vi "visualization.vi"() -> ()   [LabVIEW 2024]
uses:
  <vilib>/Analysis/baseanly.llb/Mean (DBL).vi
  <vilib>/picture/3D Picture Control/Object/Create Object (name).vi
  <vilib>/Utility/file.llb/Read Delimited Spreadsheet (string).vi
  <vilib>/picture/3D Picture Control/Helpers/Set Light (no reference).vi
  <vilib>/picture/3D Picture Control/NI_3D Picture Control.lvlib
  <vilib>/Analysis/NI_AALBase.lvlib
panel:
  out "XY Graph 4":cluster{dbl[], dbl[]}[](graph)
  out "XY Graph 3":cluster{dbl[], dbl[]}[](graph)
  out "XY Graph 2":cluster{dbl[], dbl[]}[](graph)
  out "XY Graph":cluster{dbl[], dbl[]}[](graph)
  out "Slide":u8(slide) scale=0.0..100.0
  in  "stop":bool
  out "3D Picture 2":refnum<vi>(3d-picture)
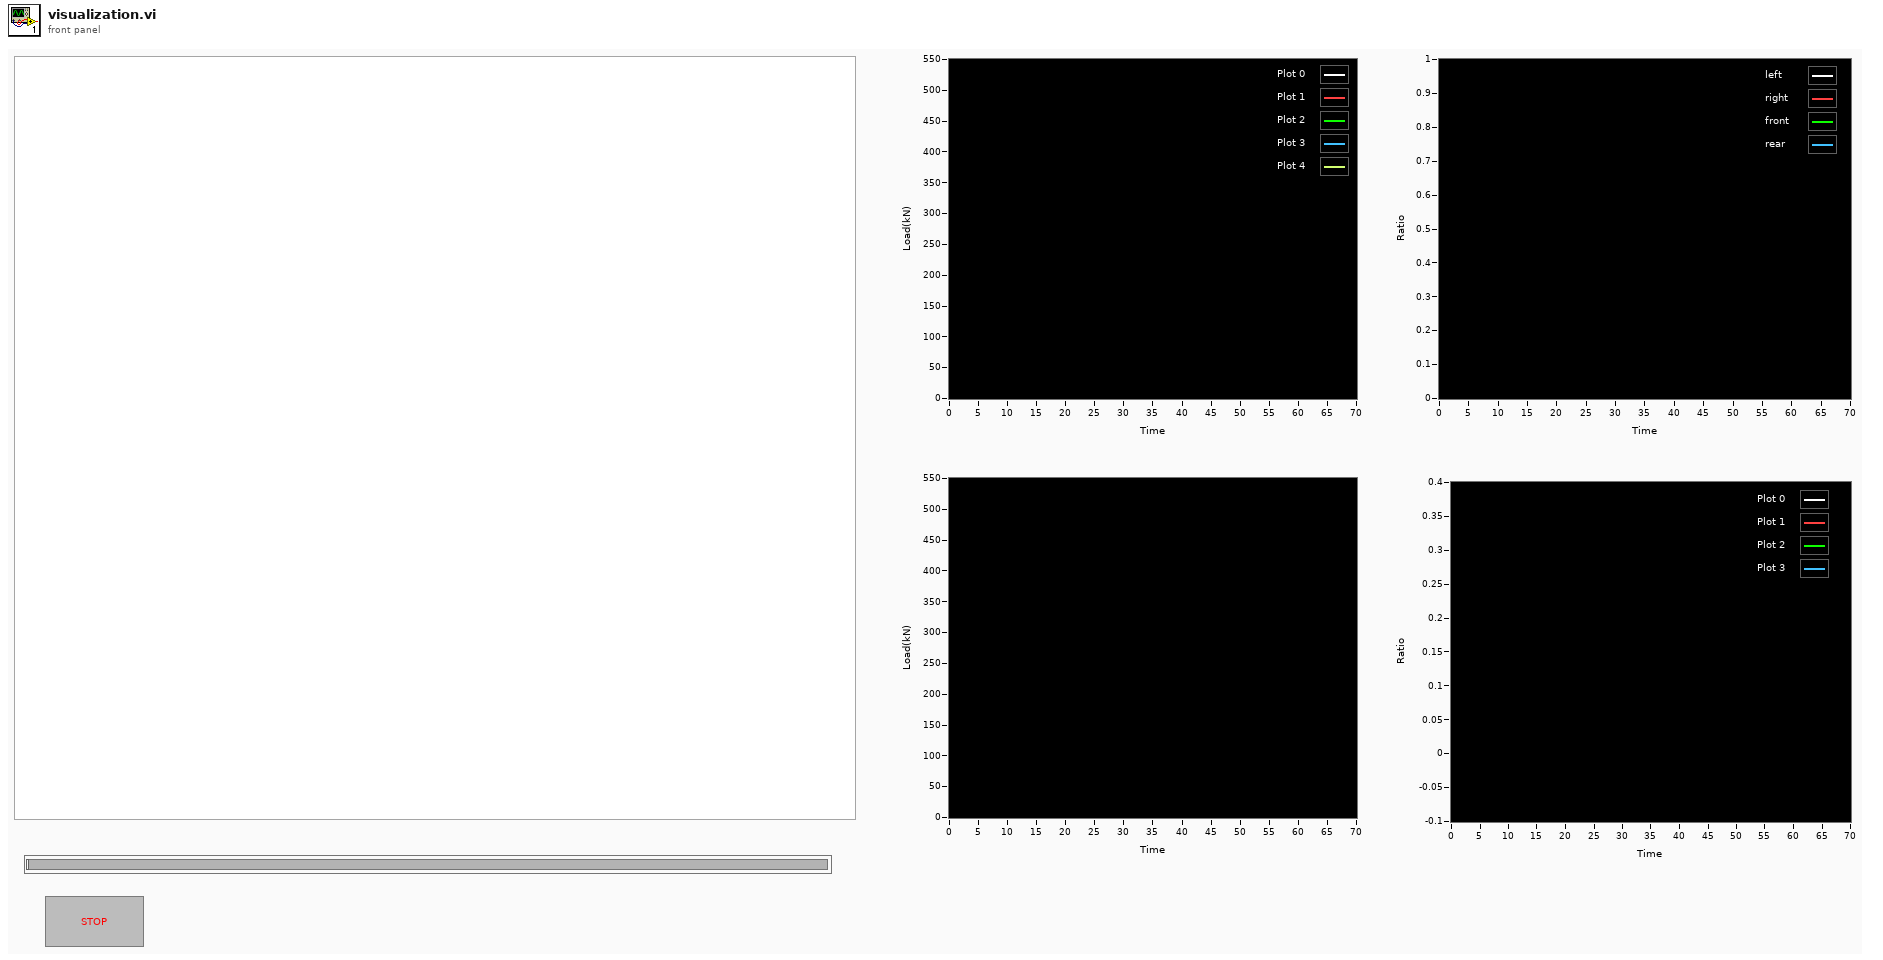
[diagram p1: front panel]
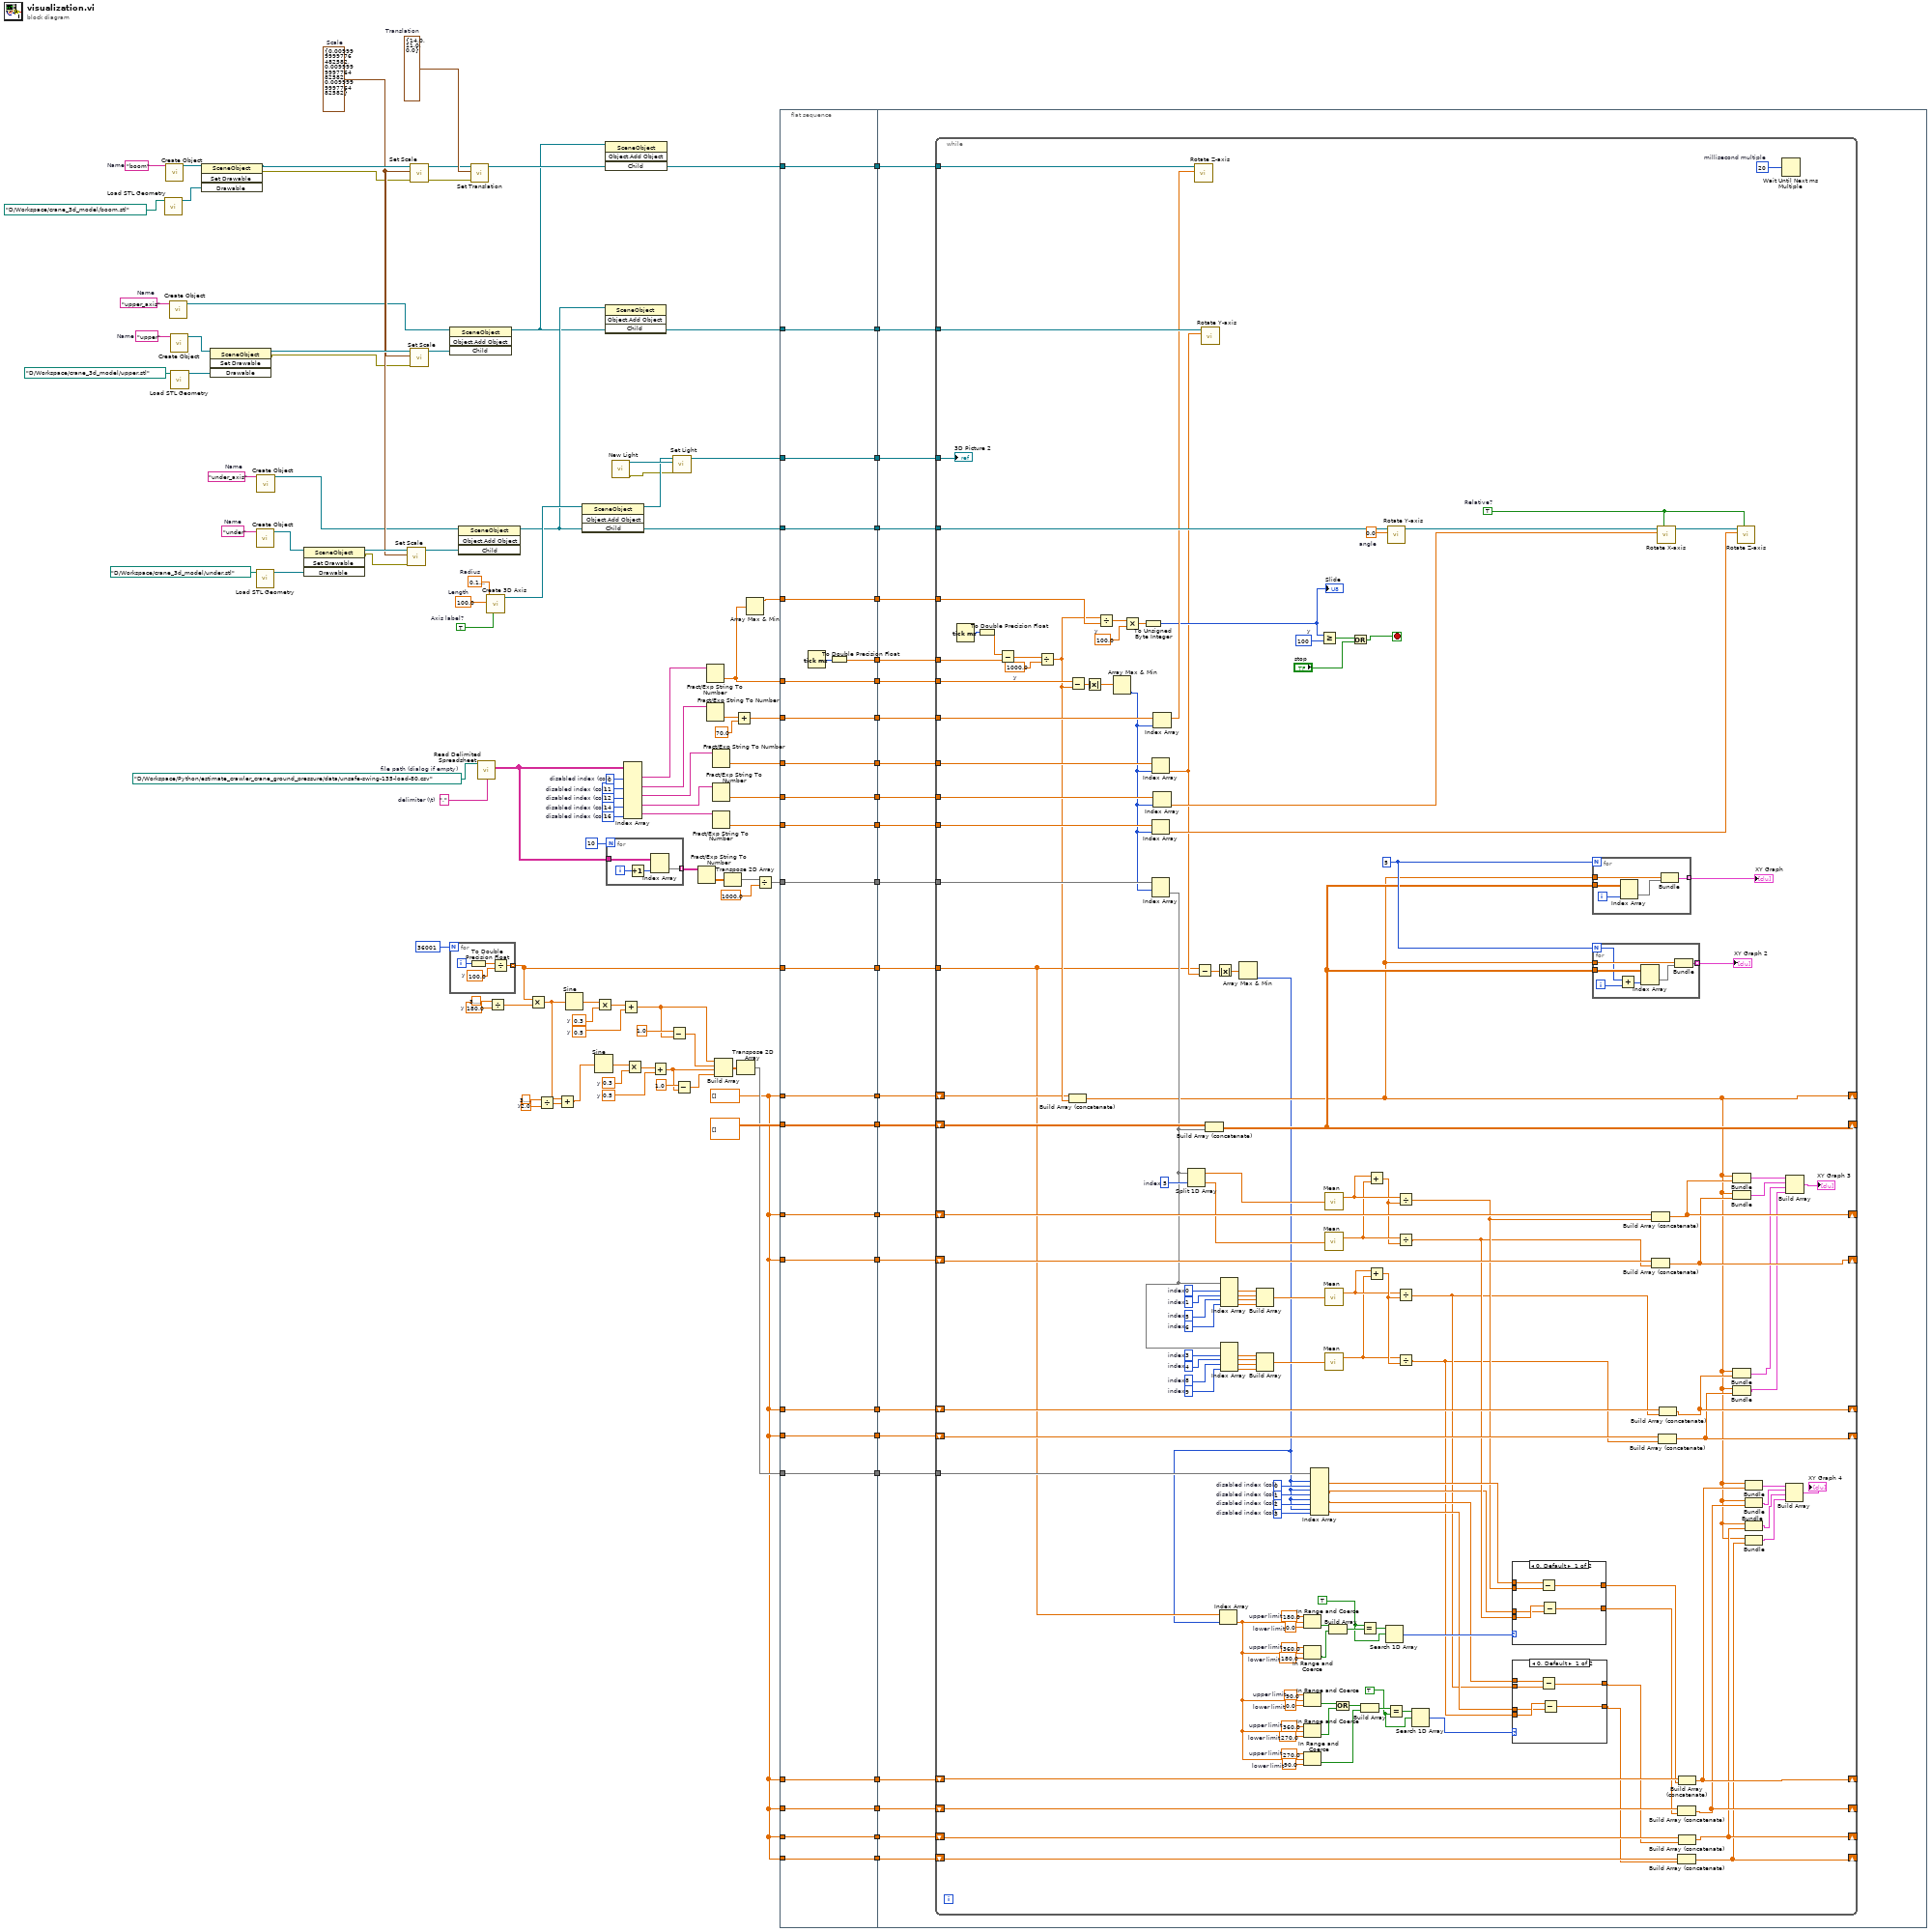
[diagram p0: block diagram]
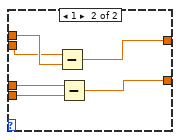
[diagram p2: hidden frame]
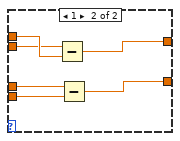
[diagram p3: hidden frame]
diagram:
  w7 = 0.5  # y
  w8 = 0.5  # y
  w15 = 0.3  # y
  w19 = 2.0  # y
  w29 = 0.3  # y
  w33 = 180.0  # y
  w1 = dbl[] []
  w66 = 16  # disabled index (col)
  w67 = 14  # disabled index (col)
  w71 = 12  # disabled index (col)
  w76 = 11  # disabled index (col)
  w77 = 0  # disabled index (col)
  w78 = ","  # delimiter (\t)
  w79 = path "D:/Workspace/Python/estimate_crawler_crane_ground_pressure/data/unsafe-swing-135-load-80.csv"  # file path (dialog if empty)
  w90 = "upper_axis"  # Name
  w92 = "under_axis"  # Name
  w102 = cluster{"X":sgl, "Y":sgl, "Z":sgl} {"X"=14.0, "Y"=11.0, "Z"=0.0}  # Translation
  w100 = cluster{"X":sgl, "Y":sgl, "Z":sgl} {"X"=0.01, "Y"=0.01, "Z"=0.01}  # Scale
  w104 = "under"  # Name
  w109 = "upper"  # Name
  w113 = sgl 0.1  # Radius
  w116 = sgl 100.0  # Length
  w118 = TRUE  # Axis label?
  w119 = "boom"  # Name
  n1 = call <vilib>:"Load STL Geometry.vi"("Model File"=path "D:/Workspace/crane_3d_model/boom.stl") -> ("New Mesh Refnum"=w117:refnum<vi>)  [unwired: 9 in, 1 out]
  n2 = call-poly <vilib>:"Create Object.vi"("Name"=w119) -> ("Scene:New Object"=w120:refnum<vi>)  [unwired: 9 in, 1 out]
  n3 = call-poly <vilib>:"Create Object.vi"("Name"=w90) -> ("Scene:New Object"=w88:refnum<vi>)  [unwired: 9 in, 1 out]
  n4 = call-poly <vilib>:"Create Object.vi"("Name"=w109) -> ("Scene:New Object"=w111:refnum<vi>)  [unwired: 9 in, 1 out]
  n5 = call <vilib>:"Load STL Geometry.vi"("Model File"=path "D:/Workspace/crane_3d_model/upper.stl") -> ("New Mesh Refnum"=w108:refnum<vi>)  [unwired: 9 in, 1 out]
  n6 = invoke class="SceneObject" method="Set Drawable"(reference=w120, "Drawable"=w117) -> (reference out=w101:refnum<vi>, error out=w99:errorcluster)  [unwired: 2 in, 2 out]
  n7 = invoke class="SceneObject" method="Set Drawable"(reference=w111, "Drawable"=w108) -> (reference out=w110:refnum<vi>, error out=w86:errorcluster)  [unwired: 2 in, 2 out]
  n8 = call-poly <vilib>:"Create Object.vi"("Name"=w104) -> ("Scene:New Object"=w105:refnum<vi>)  [unwired: 9 in, 1 out]
  n9 = call <vilib>:"Load STL Geometry.vi"("Model File"=path "D:/Workspace/crane_3d_model/under.stl") -> ("New Mesh Refnum"=w103:refnum<vi>)  [unwired: 9 in, 1 out]
  n10 = call-poly <vilib>:"Create Object.vi"("Name"=w92) -> ("Scene:New Object"=w87:refnum<vi>)  [unwired: 9 in, 1 out]
  n11 = invoke class="SceneObject" method="Set Drawable"(reference=w105, "Drawable"=w103) -> (reference out=w107:refnum<vi>, error out=w96:errorcluster)  [unwired: 2 in, 2 out]
  n12 = call <vilib>:"Set Scale.vi"("error in (no error)"=w96, "Scale"=w100, "Scene Object"=w107) -> ("Scaled Object"=w91:refnum<vi>)  [unwired: 7 in, 1 out]
  n13 = call <vilib>:"Set Scale.vi"("error in (no error)"=w99, "Scale"=w100, "Scene Object"=w101) -> ("error out"=w97:errorcluster, "Scaled Object"=w98:refnum<vi>)  [unwired: 7 in]
  n14 = call <vilib>:"Set Scale.vi"("error in (no error)"=w86, "Scale"=w100, "Scene Object"=w110) -> ("Scaled Object"=w89:refnum<vi>)  [unwired: 7 in, 1 out]
  n15 = invoke class="SceneObject" method="Object.Add Object"(reference=w88, "Child"=w89) -> (reference out=w81:refnum<vi>)  [unwired: 2 in, 3 out]
  n16 = for {
    N: 36001 -> [_]
    tunnel: [w122] -> w27 mode=indexing
    i -> [w125]
    w123 = 100.0  # y
    n17 = To Double Precision Float(number=w125) -> (double precision float=w124:dbl)
    n18 = Divide(x=w124, y=w123) -> (x/y=w122:dbl)
  }
  n19 = invoke class="SceneObject" method="Object.Add Object"(reference=w87, "Child"=w91) -> (reference out=w85:refnum<vi>)  [unwired: 2 in, 3 out]
  n20 = call <vilib>:"Set Translation.vi"("error in (no error)"=w97, "Translation"=w102, "Scene Object"=w98) -> ("Translated Object"=w82:refnum<vi>)  [unwired: 7 in, 1 out]
  n21 = call-poly <vilib>:"Read Delimited Spreadsheet.vi"("file path (dialog if empty)"=w79, "delimiter (\\t)"=w78) -> ("all rows"=w48:string[][])  [unwired: 8 in, 5 out]
  n22 = call <vilib>:"Create 3D Axis.vi"("Axis label?"=w118, "Radius"=w113, "Length"=w116) -> ("New Object Refnum"=w95:refnum<vi>)  [unwired: 7 in, 1 out]
  n23 = Divide(x=3.141592653589793, y=w33) -> (x/y=w32:dbl)
  n24 = Multiply(x=w27, y=w32) -> (x*y=w17:dbl[])
  n25 = Divide(x=3.141592653589793, y=w19) -> (x/y=w16:dbl)
  n26 = Add(x=w17, y=w16) -> (x+y=w13:dbl[])
  n27 = Sine(x=w17) -> (sin(x)=w31:dbl[])
  n28 = invoke class="SceneObject" method="Object.Add Object"(reference=w95, "Child"=w85) -> (reference out=w94:refnum<vi>, "Child"=w93:refnum<vi>)  [unwired: 2 in, 2 out]
  n29 = Sine(x=w13) -> (sin(x)=w12:dbl[])
  n30 = Multiply(x=w31, y=w29) -> (x*y=w30:dbl[])
  n31 = invoke class="SceneObject" method="Object.Add Object"(reference=w85, "Child"=w81) -> ("Child"=w84:refnum<vi>)  [unwired: 2 in, 3 out]
  n32 = invoke class="SceneObject" method="Object.Add Object"(reference=w81, "Child"=w82) -> ("Child"=w83:refnum<vi>)  [unwired: 2 in, 3 out]
  n33 = for {
    N: 10 -> [_]
    tunnel: w48 -> [w129]
    tunnel: [w126] -> w46 mode=indexing
    i -> [w128]
    n34 = Increment(x=w128) -> (x+1=w127:i32)
    n35 = Index Array "Index Array"(array=w129, index (col)=w127) -> (element=w126:string[])  [unwired: 1 in]
  }
  n36 = call <vilib>:"New Light.vi"() -> ("error out"=w80:errorcluster, "New Light Refnum"=w115:refnum<vi>)  [unwired: 10 in]
  n37 = Add(x=w30, y=w7) -> (x+y=w21:dbl[])
  n38 = Index Array "Index Array"(array=w48, index (col) #1=w77, index (col) #2=w76, index (col) #3=w71, index (col) #4=w67, index (col) #5=w66) -> (element #1=w68:string[], element #2=w69:string[], element #3=w70:string[], element #4=w65:string[], element #5=w64:string[])  [unwired: 5 in]
  n39 = Multiply(x=w12, y=w15) -> (x*y=w14:dbl[])
  n40 = Add(x=w14, y=w8) -> (x+y=w10:dbl[])
  n41 = Subtract(x=1.0, y=w21) -> (x-y=w20:dbl[])
  n42 = call-poly <vilib>:"Set Light.vi"("error in (no error)"=w80, "Light Refnum In"=w115, "Scene Object In"=w94) -> ("Scene Object Out"=w114:refnum<vi>)  [unwired: 7 in, 1 out]
  n43 = Subtract(x=1.0, y=w10) -> (x-y=w9:dbl[])
  n44 = Fract/Exp String To Number(string=w46) -> (number=w45:dbl[][])  [unwired: 3 in, 1 out]
  n45 = Fract/Exp String To Number(string=w68) -> (number=w51:dbl[])  [unwired: 3 in, 1 out]
  n46 = Fract/Exp String To Number(string=w69) -> (number=w75:dbl[])  [unwired: 3 in, 1 out]
  n47 = Fract/Exp String To Number(string=w70) -> (number=w73:dbl[])  [unwired: 3 in, 1 out]
  n48 = Fract/Exp String To Number(string=w65) -> (number=w63:dbl[])  [unwired: 3 in, 1 out]
  n49 = Fract/Exp String To Number(string=w64) -> (number=w62:dbl[])  [unwired: 3 in, 1 out]
  n50 = Build Array(w21, w20, w10, w9) -> (w5:dbl[][])
  n51 = Transpose 2D Array(2D array=w45) -> (transposed array=w40:dbl[][])
  n52 = Add(x=w75, y=70.0) -> (x+y=w72:dbl[])
  n53 = Transpose 2D Array(2D array=w5) -> (transposed array=w4:dbl[][])
  n54 = Array Max & Min(array=w51) -> (max value=w49:dbl)  [unwired: 3 out]
  n55 = Divide(x=w40, y=1000.0) -> (x/y=w39:dbl[][])
  n56 = flat-sequence {
    tunnel: w62 -> [w146]
    tunnel: w63 -> [w147]
    tunnel: w51 -> [w148]
    tunnel: w72 -> [w149]
    tunnel: w73 -> [w150]
    tunnel: w83 -> [w151]
    tunnel: w84 -> [w152]
    tunnel: w93 -> [w153]
    tunnel: w114 -> [w154]
    tunnel: [w154] -> w61
    tunnel: [w153] -> w60
    tunnel: [w152] -> w59
    tunnel: [w151] -> w58
    tunnel: [w150] -> w57
    tunnel: [w149] -> w56
    tunnel: [w148] -> w55
    tunnel: [w147] -> w54
    tunnel: [w146] -> w53
    tunnel: [w144] -> w52
    tunnel: [w143] -> w50
    tunnel: w49 -> [w143]
    tunnel: [w142] -> w44
    tunnel: w39 -> [w142]
    tunnel: [w141] -> w43
    tunnel: w1 -> [w141]
    tunnel: [w140] -> w42
    tunnel: dbl[][] [] -> [w140]
    tunnel: [w139] -> w37
    tunnel: w1 -> [w139]
    tunnel: [w138] -> w36
    tunnel: w1 -> [w138]
    tunnel: [w137] -> w28
    tunnel: w27 -> [w137]
    tunnel: [w136] -> w26
    tunnel: w1 -> [w136]
    tunnel: [w135] -> w24
    tunnel: w1 -> [w135]
    tunnel: [w134] -> w23
    tunnel: w1 -> [w134]
    tunnel: [w133] -> w22
    tunnel: w1 -> [w133]
    tunnel: [w132] -> w6
    tunnel: w4 -> [w132]
    tunnel: [w131] -> w3
    tunnel: w1 -> [w131]
    tunnel: [w130] -> w2
    tunnel: w1 -> [w130]
    tunnel: w61 -> [w178]
    tunnel: w60 -> [w177]
    tunnel: w59 -> [w176]
    tunnel: w58 -> [w175]
    tunnel: w57 -> [w174]
    tunnel: w56 -> [w173]
    tunnel: w55 -> [w172]
    tunnel: w54 -> [w171]
    tunnel: w53 -> [w170]
    tunnel: w52 -> [w169]
    tunnel: w50 -> [w168]
    tunnel: w44 -> [w167]
    tunnel: w43 -> [w166]
    tunnel: w42 -> [w165]
    tunnel: w37 -> [w164]
    tunnel: w36 -> [w163]
    tunnel: w28 -> [w162]
    tunnel: w26 -> [w161]
    tunnel: w24 -> [w160]
    tunnel: w23 -> [w159]
    tunnel: w22 -> [w158]
    tunnel: w6 -> [w157]
    tunnel: w3 -> [w156]
    tunnel: w2 -> [w155]
    frame #0 {
      n57 = Tick Count (ms)() -> (millisecond timer value=w145:u32)
      n58 = To Double Precision Float(number=w145) -> (double precision float=w144:dbl)
    }
    frame #1 {
      n59 = while {
        tunnel: w178 -> [w321]
        tunnel: w176 -> [w320]
        tunnel: w177 -> [w318]
        tunnel: w175 -> [w319]
        tunnel: w174 -> [w313]
        tunnel: w173 -> [w314]
        tunnel: w172 -> [w308]
        tunnel: w171 -> [w304]
        tunnel: w170 -> [w303]
        tunnel: w169 -> [w300]
        tunnel: w168 -> [w298]
        tunnel: w167 -> [w289]
        shift-right: [w218] -> _
        shift-left: w166 -> [w287]
        shift-right: [w282] -> _
        shift-left: w165 -> [w286]
        shift-right: [w277] -> _
        shift-left: w164 -> [w278]
        shift-right: [w273] -> _
        shift-left: w163 -> [w274]
        tunnel: w162 -> [w217]
        shift-right: [w264] -> _
        shift-left: w161 -> [w265]
        shift-right: [w225] -> _
        shift-left: w160 -> [w259]
        shift-right: [w234] -> _
        shift-left: w159 -> [w236]
        shift-right: [w233] -> _
        shift-left: w158 -> [w235]
        tunnel: w157 -> [w230]
        shift-right: [w222] -> _
        shift-left: w156 -> [w224]
        shift-right: [w219] -> _
        shift-left: w155 -> [w223]
        stop <- w290 stop-if-true
        w183 = TRUE
        w194 = 90.0  # lower limit
        w193 = 270.0  # upper limit
        w199 = 270.0  # lower limit
        w200 = 360.0  # upper limit
        w198 = 0.0  # lower limit
        w197 = 90.0  # upper limit
        w208 = TRUE
        w214 = 180.0  # lower limit
        w213 = 360.0  # upper limit
        w215 = 0.0  # lower limit
        w216 = 180.0  # upper limit
        w226 = 3  # disabled index (col)
        w227 = 2  # disabled index (col)
        w228 = 1  # disabled index (col)
        w229 = 0  # disabled index (col)
        w246 = 9  # index
        w245 = 8  # index
        w244 = 4  # index
        w243 = 3  # index
        w255 = 6  # index
        w256 = 5  # index
        w257 = 1  # index
        w258 = 0  # index
        w280 = 5  # index
        w284 = 5
        w293 = u8 100  # y
        w296 = 100.0  # y
        w299 = 0.0  # angle
        w309 = 1000.0  # y
        w315 = TRUE  # Relative?
        w322 = u32 20  # millisecond multiple
        n60 = Tick Count (ms)() -> (millisecond timer value=w312:u32)
        n61 = To Double Precision Float(number=w312) -> (double precision float=w311:dbl)
        n62 = Subtract(x=w311, y=w300) -> (x-y=w310:dbl)
        n63 = Divide(x=w310, y=w309) -> (x/y=w288:dbl)
        n64 = Build Array (concatenate)(w287, w288) -> (w218:dbl[])
        n65 = Subtract(x=w308, y=w288) -> (x-y=w307:dbl[])
        n66 = Absolute Value(x=w307) -> (abs(x)=w306:dbl[])
        n67 = Divide(x=w288, y=w298) -> (x/y=w297:dbl)
        n68 = Array Max & Min(array=w306) -> (min index (indices)=w281:i32)  [unwired: 3 out]
        n69 = Multiply(x=w297, y=w296) -> (x*y=w295:dbl)
        n70 = To Unsigned Byte Integer(number=w295) -> (unsigned 8bit integer=w294:u8)
        "Slide" <- w294
        n71 = Index Array(array=w313, index=w281) -> (element=w267:dbl)
        n72 = Index Array(array=w303, index=w281) -> (element=w301:dbl)
        n73 = Index Array(array=w289, index (row)=w281) -> (element=w242:dbl[])  [unwired: 1 in]
        n74 = Index Array(array=w314, index=w281) -> (element=w305:dbl)
        n75 = Index Array(array=w304, index=w281) -> (element=w302:dbl)
        n76 = Split 1D Array(array=w242, index=w280) -> (first subarray=w279:dbl[], second subarray=w275:dbl[])
        n77 = call <vilib>:"Rotate Z-axis.vi"("angle"=w305, "Scene Object In"=w319) -> ()  [unwired: 8 in, 2 out]
        n78 = Subtract(x=w217, y=w267) -> (x-y=w266:dbl[])
        n79 = call <vilib>:"Rotate Y-axis.vi"("angle"=w267, "Scene Object In"=w320) -> ()  [unwired: 8 in, 2 out]
        n80 = Build Array (concatenate)(w286, w242) -> (w282:dbl[][])
        n81 = Absolute Value(x=w266) -> (abs(x)=w262:dbl[])
        n82 = Index Array(array=w242, index #1=w258, index #2=w257, index #3=w256, index #4=w255) -> (element #1=w254:dbl, element #2=w253:dbl, element #3=w252:dbl, element #4=w251:dbl)
        n83 = Index Array(array=w242, index #1=w243, index #2=w244, index #3=w245, index #4=w246) -> (element #1=w247:dbl, element #2=w248:dbl, element #3=w249:dbl, element #4=w250:dbl)
        n84 = Array Max & Min(array=w262) -> (min index (indices)=w189:i32)  [unwired: 3 out]
        n85 = Index Array(array=w217, index=w189) -> (element=w179:dbl)
        n86 = Build Array(w254, w253, w252, w251) -> (w241:dbl[])
        n87 = Build Array(w247, w248, w249, w250) -> (w240:dbl[])
        n88 = In Range and Coerce(upper limit=w216, x=w179, lower limit=w215) -> (In Range?=w212:bool)  [unwired: 1 out]
        n89 = In Range and Coerce(upper limit=w213, x=w179, lower limit=w214) -> (In Range?=w211:bool)  [unwired: 1 out]
        n90 = In Range and Coerce(upper limit=w197, x=w179, lower limit=w198) -> (In Range?=w196:bool)  [unwired: 1 out]
        n91 = In Range and Coerce(upper limit=w200, x=w179, lower limit=w199) -> (In Range?=w195:bool)  [unwired: 1 out]
        n92 = In Range and Coerce(upper limit=w193, x=w179, lower limit=w194) -> (In Range?=w191:bool)  [unwired: 1 out]
        n93 = Index Array "Index Array"(array=w230, index (row) #1=w189, index (col) #1=w229, index (row) #2=w189, index (col) #2=w228, index (row) #3=w189, index (col) #3=w227, index (row) #4=w189, index (col) #4=w226) -> (element #1=w206:dbl, element #2=w203:dbl, element #3=w188:dbl, element #4=w187:dbl)
        n94 = Greater Or Equal?(x=w294, y=w293) -> (x >= y?=w292:bool)
        n95 = call-poly <vilib>:"Mean.vi"("X"=w279) -> ("mean"=w270:dbl)  [unwired: 1 out]
        n96 = call-poly <vilib>:"Mean.vi"("X"=w275) -> ("mean"=w269:dbl)  [unwired: 1 out]
        n97 = call-poly <vilib>:"Mean.vi"("X"=w241) -> ("mean"=w238:dbl)  [unwired: 1 out]
        n98 = call-poly <vilib>:"Mean.vi"("X"=w240) -> ("mean"=w237:dbl)  [unwired: 1 out]
        n99 = Build Array(w212, w211) -> (w210:bool[])
        n100 = Or(x=w196, y=w195) -> (x .or. y?=w192:bool)
        n101 = Or(x=w292, y="stop") -> (x .or. y?=w290:bool)
        n102 = Equal?(x=w208, y=w210) -> (x = y?=w209:bool[])
        n103 = Build Array(w192, w191) -> (w190:bool[])
        n104 = Add(x=w270, y=w269) -> (x+y=w268:dbl)
        n105 = Add(x=w238, y=w237) -> (x+y=w239:dbl)
        n106 = Search 1D Array(1D array=w209, element=w208) -> (index of element=w207:i32)  [unwired: 1 in]
        n107 = call <vilib>:"Rotate Y-axis.vi"("angle"=w299, "Scene Object In"=w318) -> ("Scene Object Out"=w317:refnum<vi>)  [unwired: 8 in, 1 out]
        n108 = Equal?(x=w190, y=w183) -> (x = y?=w184:bool[])
        n109 = Divide(x=w270, y=w268) -> (x/y=w205:dbl)
        n110 = Divide(x=w269, y=w268) -> (x/y=w204:dbl)
        n111 = Divide(x=w238, y=w239) -> (x/y=w186:dbl)
        n112 = Divide(x=w237, y=w239) -> (x/y=w185:dbl)
        n113 = Search 1D Array(1D array=w184, element=w183) -> (index of element=w182:i32)  [unwired: 1 in]
        n114 = case shown="0, Default" w207 {
          tunnel: w206 -> [w340 w346]
          tunnel: w205 -> [w339 w345]
          tunnel: w204 -> [w337 w343]
          tunnel: w203 -> [w336 w342]
          tunnel: [w338 w344] -> w202
          tunnel: [w335 w341] -> w201
          frame 0, Default {
            n115 = Subtract(x=w340, y=w339) -> (x-y=w338:dbl)
            n116 = Subtract(x=w337, y=w336) -> (x-y=w335:dbl)
          }
          frame 1 {
            n117 = Subtract(x=w345, y=w346) -> (x-y=w344:dbl)
            n118 = Subtract(x=w342, y=w343) -> (x-y=w341:dbl)
          }
        }
        n119 = case shown="0, Default" w182 {
          tunnel: w188 -> [w328 w334]
          tunnel: w186 -> [w327 w333]
          tunnel: w185 -> [w325 w331]
          tunnel: w187 -> [w324 w330]
          tunnel: [w326 w332] -> w181
          tunnel: [w323 w329] -> w180
          frame 0, Default {
            n120 = Subtract(x=w328, y=w327) -> (x-y=w326:dbl)
            n121 = Subtract(x=w325, y=w324) -> (x-y=w323:dbl)
          }
          frame 1 {
            n122 = Subtract(x=w333, y=w334) -> (x-y=w332:dbl)
            n123 = Subtract(x=w330, y=w331) -> (x-y=w329:dbl)
          }
        }
        n124 = for {
          N: w284 -> [_]
          tunnel: w218 -> [w358]
          tunnel: w282 -> [w356]
          tunnel: [w357] -> w285 mode=indexing
          i -> [w355]
          n125 = Index Array(array=w356, index (col)=w355) -> (element=w354:dbl[])  [unwired: 1 in]
          n126 = Bundle(w358, w354) -> (w357:cluster{dbl[], dbl[]})  [unwired: 1 in]
        }
        "XY Graph" <- w285
        n127 = for {
          N: w284 -> [w347]
          tunnel: w218 -> [w353]
          tunnel: w282 -> [w351]
          tunnel: [w352] -> w283 mode=indexing
          i -> [w350]
          n128 = Add(x=w347, y=w350) -> (x+y=w348:i32)
          n129 = Index Array(array=w351, index (col)=w348) -> (element=w349:dbl[])  [unwired: 1 in]
          n130 = Bundle(w353, w349) -> (w352:cluster{dbl[], dbl[]})  [unwired: 1 in]
        }
        "XY Graph 2" <- w283
        n131 = Build Array (concatenate)(w278, w205) -> (w277:dbl[])
        n132 = Build Array (concatenate)(w274, w204) -> (w273:dbl[])
        n133 = call <vilib>:"Rotate X-axis.vi"("Relative?"=w315, "angle"=w302, "Scene Object In"=w317) -> ("Scene Object Out"=w316:refnum<vi>)  [unwired: 7 in, 1 out]
        n134 = Build Array (concatenate)(w235, w185) -> (w233:dbl[])
        n135 = Build Array (concatenate)(w236, w186) -> (w234:dbl[])
        n136 = Build Array (concatenate)(w259, w201) -> (w225:dbl[])
        n137 = Build Array (concatenate)(w223, w180) -> (w219:dbl[])
        n138 = Build Array (concatenate)(w265, w202) -> (w264:dbl[])
        n139 = Build Array (concatenate)(w224, w181) -> (w222:dbl[])
        n140 = Bundle(w218, w277) -> (w276:cluster{dbl[], dbl[]})  [unwired: 1 in]
        n141 = Bundle(w218, w273) -> (w271:cluster{dbl[], dbl[]})  [unwired: 1 in]
        n142 = Bundle(w218, w234) -> (w232:cluster{dbl[], dbl[]})  [unwired: 1 in]
        n143 = Bundle(w218, w233) -> (w231:cluster{dbl[], dbl[]})  [unwired: 1 in]
        n144 = call <vilib>:"Rotate Z-axis.vi"("Relative?"=w315, "angle"=w301, "Scene Object In"=w316) -> ()  [unwired: 7 in, 2 out]
        n145 = Bundle(w218, w264) -> (w263:cluster{dbl[], dbl[]})  [unwired: 1 in]
        n146 = Bundle(w218, w225) -> (w260:cluster{dbl[], dbl[]})  [unwired: 1 in]
        n147 = Bundle(w218, w222) -> (w221:cluster{dbl[], dbl[]})  [unwired: 1 in]
        n148 = Bundle(w218, w219) -> (w220:cluster{dbl[], dbl[]})  [unwired: 1 in]
        n149 = Wait Until Next ms Multiple(millisecond multiple=w322) -> ()  [unwired: 1 out]
        n150 = Build Array(w263, w260, w221, w220) -> (→"XY Graph 4":cluster{dbl[], dbl[]}[])
        n151 = Build Array(w276, w271, w232, w231) -> (→"XY Graph 3":cluster{dbl[], dbl[]}[])
        "3D Picture 2" <- w321
      }
    }
  }
